vi "reset.vi"(8 "error in (no error)":errorcluster, 11 "DmmKeysight in":refnum<class "DmmKeysight.lvclass">) -> (0 "error out":errorcluster, 3 "DmmKeysight out":refnum<class "DmmKeysight.lvclass">)   [LabVIEW 2023, in "DmmKeysight.lvclass"]
doc: "<b>Author:</b> Wolfgang\n<b>Description:</b> This method is used to reset the instrument to a default and known state."
uses:
  DmmKeysight.lvclass
  DmmKeysight.lvclass/DmmKeysight.ctl
  Driver/Keysight-34450A.lvlib
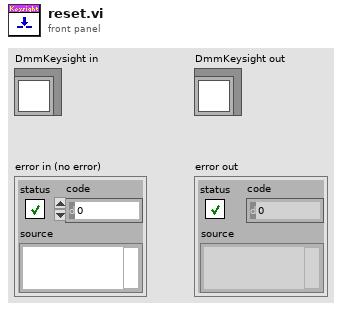
[diagram p1: front panel]
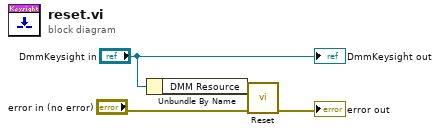
[diagram p0: block diagram]
diagram:
  n1 = Unbundle By Name("DmmKeysight in") -> ("DMM Resource"=w4:refnum<visa-resource-name>)
  n2 = call "Reset.vi"("error in (no error)"="error in (no error)", "VISA resource name"=w4) -> ("error out"=→"error out":errorcluster)  [unwired: 8 in, 1 out]
  "DmmKeysight out" <- "DmmKeysight in"
